vi "hse-application_ApplicationShutdown.vi"(8 "error in":errorcluster) -> (0 "error out":errorcluster)   [LabVIEW 2022 SP3, in "hse-application.lvclass"]
doc: "Stops and frees all hse resources.\n\n\n\n____\nHAMPEL SOFTWARE ENGINEERING v3.8.0 (2023-12-18 14:41)"
uses:
  hse-application.lvclass
  hse-application.lvclass/hse-application.ctl
  <vilib>/event_ctls.llb/usereventprio.ctl
  hse-misc/Error/Error_Labels.ctl
  <vilib>/Utility/error.llb/Error Cluster From Error Code.vi
  hse-misc/Error/Error_Helper_RaiseErrorFromLabel.vi
  hse-misc/hse-misc.lvlib
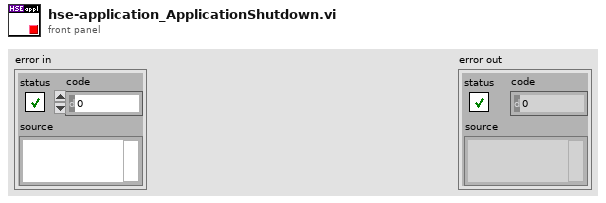
[diagram p1: front panel]
types:
  T1 = typedef "usereventprio.ctl" = enum32{"high priority", "normal priority"}
  T2 = typedef "hse-misc.lvlib/Error_Labels.ctl" = enum16{"=== GENERIC ===", "Unexpected / unknown error", "Timeout", "Device or resource not found", "Expected (handled) error", "Module or VI not executable", "Server shutting down", "File not found", "Cancelled by user", "Invalid parameter", "Configuration type invalid", "Configuration token not found", "Error occurred parsing configuration string", "External program returned with error", "Unexpected data", "Unknown message", "Attribute not found (in a variant or tree)", "Number of elements mismatch (e.g. in an array)", "Maximum number of attempts (e.g. for a reconnection)", "Input out of range", "Registry file not found or not readable", "Registry type mismatch", "Project name mismatch", "System identifier mismatch", "Configuration file not found", "Checking remote path failed", "Establishing data connection failed", "The network operation exceeded the time limit", "Network is down/unreachable/reset", "The specified port or network address is currently in use", "=== NI DISCOVERY PROTOCOL ===", "=== APPLICATION BUILDER ===", "=== GIT ===", "Return code != 0", "=== FGPA ===", "Generic FPGA error", "Timeout general", "Timeout FIFO", "Timeout DMA", "Timeout Handshake", "Loop time exceeded", "=== IO ===", "=== PROFINET ===", "=== USER INTERFACE ===", "=== GENERIC NETWORKING (NET-TX & NET-RX ==="}
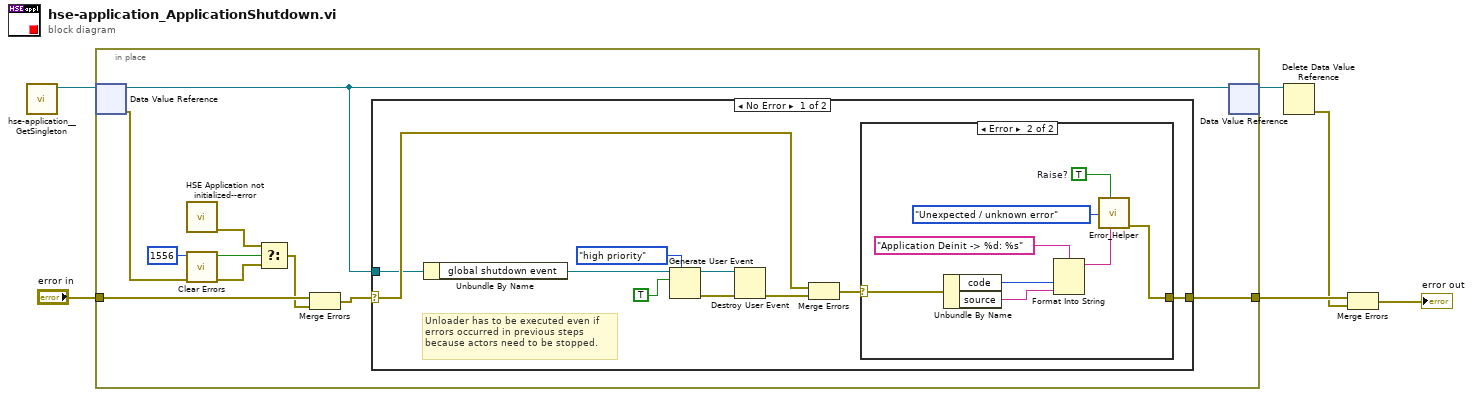
[diagram p0: block diagram]
diagram:
  n1 = call "hse-application__GetSingleton.vi"() -> ("ApplicationClass DVR"=w5:refnum<data-value>)  [unwired: 10 in, 1 out]
  n2 = in-place "In Place Element Structure" {
    in-place-border: "error in" -> [w16]
    in-place-border: [w15] -> w3
    n3 = in-place-dvr #1(w5) -> (w14:refnum<class "hse-application.lvclass">, w9:errorcluster)
    n4 = call "HSE Application not initialized--error.vi"() -> ("error out"=w11:errorcluster)  [unwired: 11 in]
    n5 = call <vilib>:"Clear Errors.vi"("error in (no error)"=w9, "specific error code to clear (0: all)"=1556) -> ("error out"=w10:errorcluster, "specific error cleared?"=w12:bool)  [unwired: 4 in]
    n6 = Select(t=w11, s=w12, f=w10) -> (s? t:f=w7:errorcluster)
    n7 = Merge Errors(w16, w7) -> (w8:errorcluster)
    n8 = case shown="No Error" w8 {
      selector: w8 -> [w25 w36]
      tunnel: [w24 w36] -> w15
      tunnel: w14 -> [w23 _]
      frame No Error {
        # "Unloader has to be executed even if \nerrors occurred in previous steps \nbecause actors need to be stopped."
        n9 = Unbundle By Name(w23) -> ("global shutdown event"=w22:refnum<user-event>)
        n10 = Generate User Event(priority (normal)=usereventprio."high priority", user event=w22, event data cluster=TRUE ("event data")) -> (user event out=w19:refnum<user-event>, error out=w18:errorcluster)  [unwired: 1 in]
        n11 = Destroy User Event(user event=w19, error in=w18) -> (error out=w17:errorcluster)
        n12 = Merge Errors(w25, w17) -> (w26:errorcluster)
        n13 = case shown="Error" w26 {
          selector: w26 -> [w27 w31]
          tunnel: [w27 w30] -> w24
          frame No Error {
          }
          frame Error {
            w29 = TRUE  # Raise?
            n14 = Unbundle By Name(w31) -> ("code"=w35:i32, "source"=w34:string)
            n15 = Format Into String(format string="Application Deinit -> %d: %s", w35, w34) -> (resulting string=w32:string)  [unwired: 2 in, 1 out]
            n16 = call-poly "Error_Helper.vi"("Additional Info"=w32, "Raise?"=w29, "Error Labels"=Error_Labels."Unexpected / unknown error") -> ("Error Out"=w30:errorcluster)  [unwired: 8 in]
          }
        }
      }
      frame Error {
      }
    }
    n17 = in-place-dvr #1(w14) -> (w4:refnum<data-value>)  [unwired: 1 out]
  }
  n18 = Delete Data Value Reference(data value reference=w4) -> (error out=w2:errorcluster)  [unwired: 1 in, 1 out]
  n19 = Merge Errors(w3, w2) -> (→"error out":errorcluster)
